vi "updateDomainMetadata.vi"(8 "error in":errorcluster, 11 "IDataDescriptor in":refnum<class "IDataDescriptor.lvclass">) -> (0 "error out":errorcluster, 3 "IDataDescriptor out":refnum<class "IDataDescriptor.lvclass">)   [LabVIEW 2022 SP3, in "openDAQ.lvlib" / "daqUtils.lvlib"]
uses:
  daqUtils.lvlib
  IDataDescriptor/IDataDescriptor.lvclass
  IDataRule/IDataRule.lvclass
  IUnit/IUnit.lvclass
  IBaseObject/IBaseObject.lvclass
  daqCoreTypes/IRatio/IRatio.lvclass
  daqCoreTypes/IDict/IDict.lvclass
  IBaseObject/Polymorphic/queryInterface/queryNumberInterface.vi
  daqCoreTypes/INumber/INumber.lvclass
  IReferenceDomainInfo/IReferenceDomainInfo.lvclass
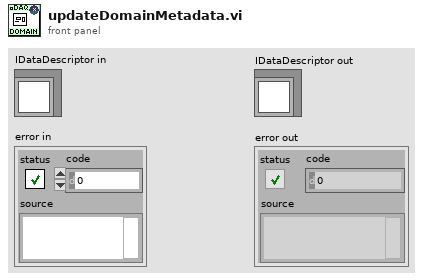
[diagram p1: front panel]
types:
  T1 = enum16{"init", "read", "set sampleRate", "set ruleStart", "set ruleDelta", "set referenceDomainOffset", "set origin", "set unitSymbol", "set resNum", "set resDen", " calculate sampleRate"}
  T2 = typedef "openDAQ.lvlib/IBaseObject.lvlib/IDataRule.lvlib/IDataRule.lvclass/DataRuleType.ctl" = u16
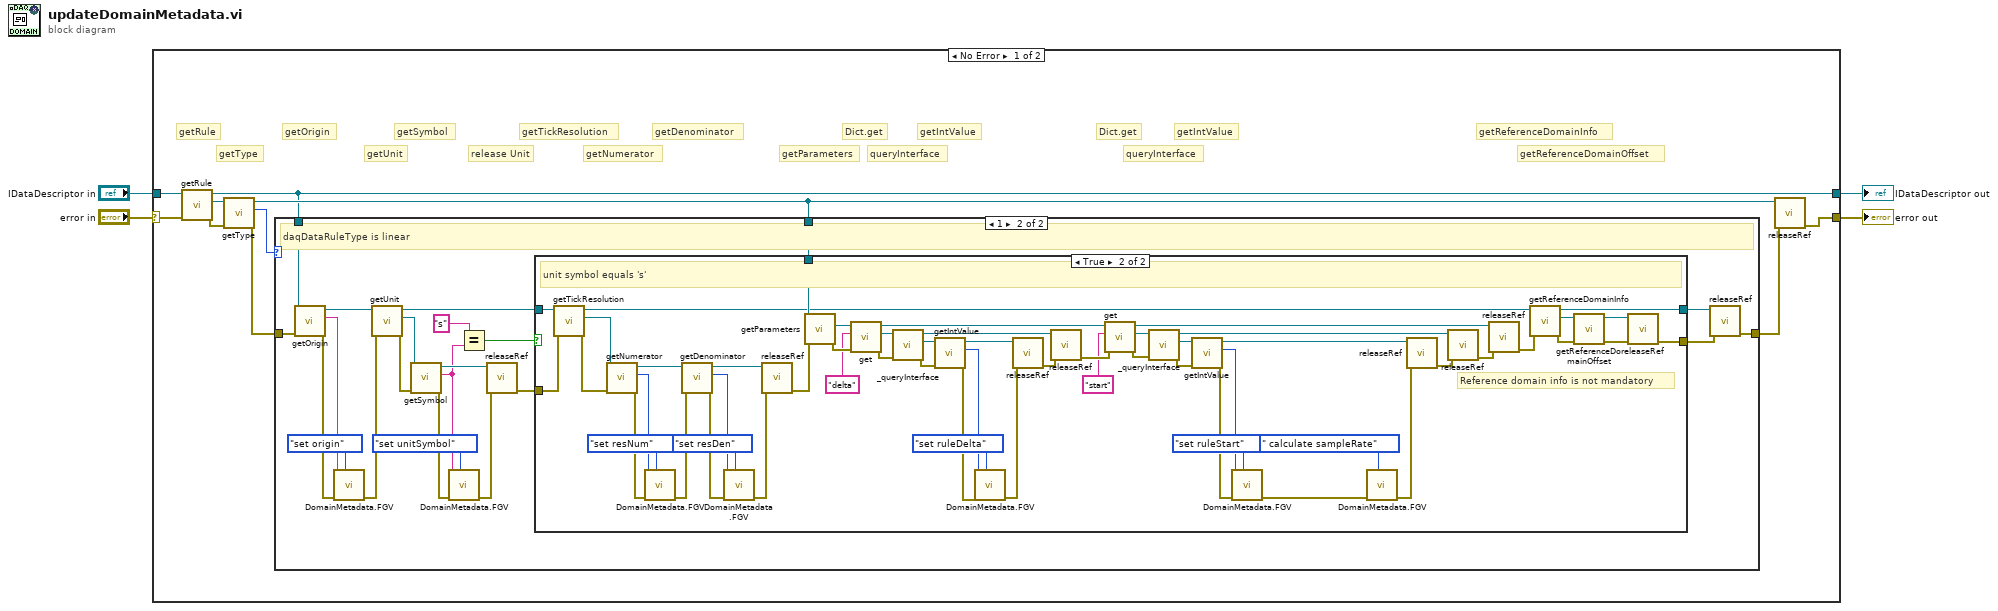
[diagram p0: block diagram]
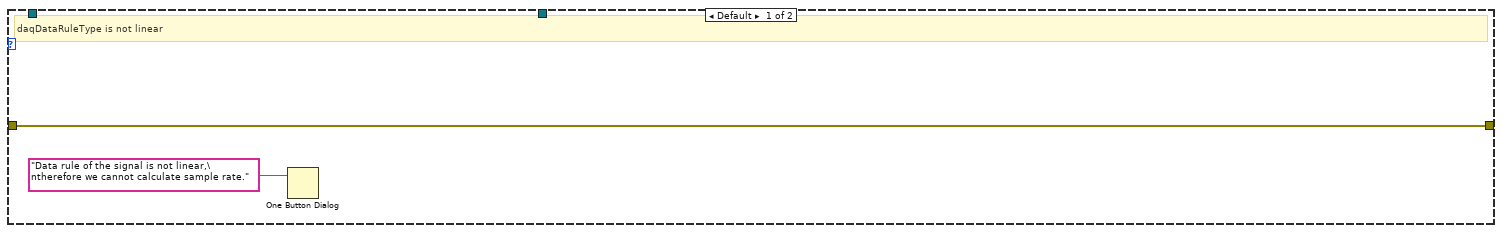
[diagram p2: hidden frame]
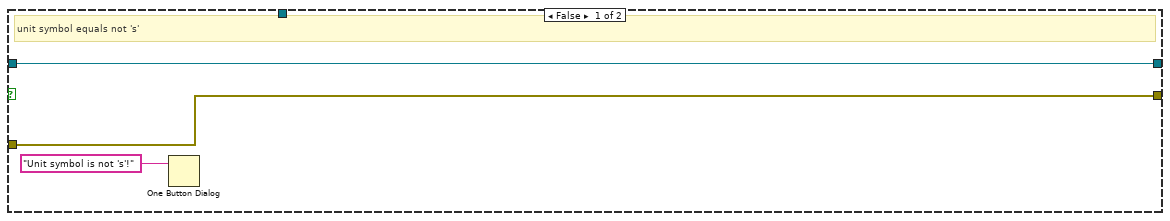
[diagram p3: hidden frame]
diagram:
  n1 = case shown="No Error" "error in" {
    selector: "error in" -> [w8 w99]
    tunnel: "IDataDescriptor in" -> [w7 w98]
    tunnel: [w5 w99] -> w1
    tunnel: [w6 w98] -> w2
    frame No Error {
      # "getRule"
      # "getType"
      # "getReferenceDomainOffset"
      # "queryInterface"
      # "queryInterface"
      # "getParameters"
      # "getNumerator"
      # "release Unit"
      # "getUnit"
      # "getReferenceDomainInfo"
      # "getIntValue"
      # "Dict.get"
      # "getIntValue"
      # "Dict.get"
      # "getDenominator"
      # "getTickResolution"
      # "getSymbol"
      # "getOrigin"
      n2 = call "getRule.vi"("error in (no error)"=w8, "IDataDescriptor in"=w7) -> ("error out"=w14:errorcluster, "DataRule out"=w13:refnum<class "IDataRule.lvclass">, "IDataDescriptor out"=w6:refnum<class "IDataDescriptor.lvclass">)  [unwired: 7 in]
      n3 = call "getType.vi"("error in (no error)"=w14, "IDataRule in"=w13) -> ("error out"=w11:errorcluster, "DataRuleType"=w12:T2, "IDataRule out"=w10:refnum<class "IDataRule.lvclass">)  [unwired: 7 in]
      n4 = case shown="1" w12 {
        tunnel: w6 -> [_ w38]
        tunnel: w11 -> [w16 w37]
        tunnel: [w16 w32] -> w9
        tunnel: w10 -> [_ w26]
        frame Default {
          # "daqDataRuleType is not linear"
          n5 = One Button Dialog(message="Data rule of the signal is not linear,\ntherefore we cannot calculate sample rate." ("modulePath")) -> ()  [unwired: 1 in, 1 out]
        }
        frame 1 {
          # "daqDataRuleType is linear"
          n6 = call "getOrigin.vi"("error in (no error)"=w37, "IDataDescriptor in"=w38) -> ("error out"=w24:errorcluster, "Origin out"=w22:string, "IDataDescriptor out"=w36:refnum<class "IDataDescriptor.lvclass">)  [unwired: 7 in]
          n7 = call "DomainMetadata.FGV.vi"("Case Select"=T1."set origin", "error in"=w24, "String in"=w22) -> ("error out"=w23:errorcluster)  [unwired: 7 in, 1 out]
          n8 = call "getUnit.vi"("error in (no error)"=w23, "IDataDescriptor in"=w36) -> ("error out"=w35:errorcluster, "Unit out"=w34:refnum<class "IUnit.lvclass">, "IDataDescriptor out"=w28:refnum<class "IDataDescriptor.lvclass">)  [unwired: 7 in]
          n9 = call "getSymbol.vi"("error in (no error)"=w35, "IUnit in"=w34) -> ("error out"=w20:errorcluster, "Symbol out"=w18:string, "IUnit out"=w33:refnum<class "IUnit.lvclass">)  [unwired: 7 in]
          n10 = call "DomainMetadata.FGV.vi"("Case Select"=T1."set unitSymbol", "error in"=w20, "String in"=w18) -> ("error out"=w19:errorcluster)  [unwired: 7 in, 1 out]
          n11 = Equal?(x="s" ("y"), y=w18) -> (x = y?=w31:bool)
          n12 = call-dynamic "releaseRef.vi"("error in (no error)"=w19, "IBaseObject in"=w33) -> ("error out"=w30:errorcluster)  [unwired: 9 in]
          n13 = case shown="True" w31 {
            tunnel: w30 -> [w41 w95]
            tunnel: [w41 w42] -> w29
            tunnel: w28 -> [w39 w96]
            tunnel: [w39 w48] -> w27
            tunnel: w26 -> [_ w89]
            frame False {
              # "unit symbol equals not 's'"
              n14 = One Button Dialog(message="Unit symbol is not 's'!") -> ()  [unwired: 1 in, 1 out]
            }
            frame True {
              # "Reference domain info is not mandatory"
              # "unit symbol equals 's'"
              n15 = call "getTickResolution.vi"("error in (no error)"=w95, "IDataDescriptor in"=w96) -> ("error out"=w94:errorcluster, "TickResolution out"=w93:refnum<class "IRatio.lvclass">, "IDataDescriptor out"=w49:refnum<class "IDataDescriptor.lvclass">)  [unwired: 7 in]
              n16 = call "getNumerator.vi"("error in (no error)"=w94, "IRatio in"=w93) -> ("error out"=w66:errorcluster, "Numerator out"=w64:i64, "IRatio out"=w92:refnum<class "IRatio.lvclass">)  [unwired: 7 in]
              n17 = call "DomainMetadata.FGV.vi"("Case Select"=T1."set resNum", "error in"=w66, "Int in"=w64) -> ("error out"=w65:errorcluster)  [unwired: 7 in, 1 out]
              n18 = call "getDenominator.vi"("error in (no error)"=w65, "IRatio in"=w92) -> ("error out"=w62:errorcluster, "Denominator out"=w61:i64, "IRatio out"=w91:refnum<class "IRatio.lvclass">)  [unwired: 7 in]
              n19 = call "DomainMetadata.FGV.vi"("Case Select"=T1."set resDen", "error in"=w62, "Int in"=w61) -> ("error out"=w60:errorcluster)  [unwired: 7 in, 1 out]
              n20 = call-dynamic "releaseRef.vi"("error in (no error)"=w60, "IBaseObject in"=w91) -> ("error out"=w90:errorcluster)  [unwired: 9 in]
              n21 = call "getParameters.vi"("error in (no error)"=w90, "IDataRule in"=w89) -> ("error out"=w87:errorcluster, "Parameters out"=w88:refnum<class "IDict.lvclass">)  [unwired: 7 in, 1 out]
              n22 = call "get.vi"("error in (no error)"=w87, "Key in"="delta" ("y"), "IDict in"=w88) -> ("error out"=w82:errorcluster, "Value out"=w83:refnum<class "IBaseObject.lvclass">, "IDict out"=w84:refnum<class "IDict.lvclass">)  [unwired: 6 in]
              n23 = call-poly "_queryInterface.vi"("error in (no error)"=w82, "IBaseObject in"=w83) -> ("error out"=w79:errorcluster, "INumber out"=w80:refnum<class "INumber.lvclass">, "IBaseObject out"=w81:refnum<class "IBaseObject.lvclass">)  [unwired: 7 in]
              n24 = call "getIntValue.vi"("error in (no error)"=w79, "INumber in"=w80) -> ("error out"=w58:errorcluster, "Int Value out"=w56:i64, "INumber out"=w71:refnum<class "INumber.lvclass">)  [unwired: 7 in]
              n25 = call "DomainMetadata.FGV.vi"("Case Select"=T1."set ruleDelta", "error in"=w58, "Int in"=w56) -> ("error out"=w57:errorcluster)  [unwired: 7 in, 1 out]
              n26 = call-dynamic "releaseRef.vi"("error in (no error)"=w57, "IBaseObject in"=w71) -> ("error out"=w70:errorcluster)  [unwired: 9 in]
              n27 = call-dynamic "releaseRef.vi"("error in (no error)"=w70, "IBaseObject in"=w81) -> ("error out"=w97:errorcluster)  [unwired: 9 in]
              n28 = call "get.vi"("error in (no error)"=w97, "Key in"="start" ("y"), "IDict in"=w84) -> ("error out"=w74:errorcluster, "Value out"=w75:refnum<class "IBaseObject.lvclass">, "IDict out"=w73:refnum<class "IDict.lvclass">)  [unwired: 6 in]
              n29 = call-poly "_queryInterface.vi"("error in (no error)"=w74, "IBaseObject in"=w75) -> ("error out"=w78:errorcluster, "INumber out"=w77:refnum<class "INumber.lvclass">, "IBaseObject out"=w76:refnum<class "IBaseObject.lvclass">)  [unwired: 7 in]
              n30 = call "getIntValue.vi"("error in (no error)"=w78, "INumber in"=w77) -> ("error out"=w53:errorcluster, "Int Value out"=w54:i64, "INumber out"=w69:refnum<class "INumber.lvclass">)  [unwired: 7 in]
              n31 = call "DomainMetadata.FGV.vi"("Case Select"=T1."set ruleStart", "error in"=w53, "Int in"=w54) -> ("error out"=w52:errorcluster)  [unwired: 7 in, 1 out]
              n32 = call "DomainMetadata.FGV.vi"("Case Select"=T1." calculate sampleRate", "error in"=w52) -> ("error out"=w51:errorcluster)  [unwired: 8 in, 1 out]
              n33 = call-dynamic "releaseRef.vi"("error in (no error)"=w51, "IBaseObject in"=w69) -> ("error out"=w68:errorcluster)  [unwired: 9 in]
              n34 = call-dynamic "releaseRef.vi"("error in (no error)"=w68, "IBaseObject in"=w76) -> ("error out"=w72:errorcluster)  [unwired: 9 in]
              n35 = call-dynamic "releaseRef.vi"("error in (no error)"=w72, "IBaseObject in"=w73) -> ("error out"=w47:errorcluster)  [unwired: 9 in]
              n36 = call "getReferenceDomainInfo.vi"("error in (no error)"=w47, "IDataDescriptor in"=w49) -> ("error out"=w45:errorcluster, "ReferenceDomainInfo out"=w46:refnum<class "IReferenceDomainInfo.lvclass">, "IDataDescriptor out"=w48:refnum<class "IDataDescriptor.lvclass">)  [unwired: 7 in]
              n37 = call "getReferenceDomainOffset.vi"("error in (no error)"=w45, "IReferenceDomainInfo in"=w46) -> ("error out"=w43:errorcluster, "IReferenceDomainInfo out"=w44:refnum<class "IReferenceDomainInfo.lvclass">)  [unwired: 7 in, 1 out]
              n38 = call-dynamic "releaseRef.vi"("error in (no error)"=w43, "IBaseObject in"=w44) -> ("error out"=w42:errorcluster)  [unwired: 9 in]
            }
          }
          n39 = call-dynamic "releaseRef.vi"("error in (no error)"=w29, "IBaseObject in"=w27) -> ("error out"=w32:errorcluster)  [unwired: 9 in]
        }
      }
      n40 = call-dynamic "releaseRef.vi"("error in (no error)"=w9, "IBaseObject in"=w10) -> ("error out"=w5:errorcluster)  [unwired: 9 in]
    }
    frame Error {
    }
  }
  "IDataDescriptor out" <- w2
  "error out" <- w1
